vi "TS DAC Acq Stop.vi"(8 "error in (no error)":errorcluster, 11 "LNG Boiling Test Stand in":refnum<class "LNG Boiling Test Stand.lvclass">) -> (0 "error out":errorcluster, 3 "LNG Boiling Test Stand out":refnum<class "LNG Boiling Test Stand.lvclass">)   [LabVIEW 2019, in "Test Stands.lvlib" / "LNG Boiling Test Stand.lvclass"]
uses:
  LNG Boiling Test Stand.lvclass
  LNG Boiling Test Stand.lvclass/LNG Boiling Test Stand.ctl
  <vilib>/DAQmx/write.llb/DAQmx Write (Analog DBL 1Chan 1Samp).vi
  <vilib>/DAQmx/miscellaneous.llb/DAQmx Fill In Error Info.vi
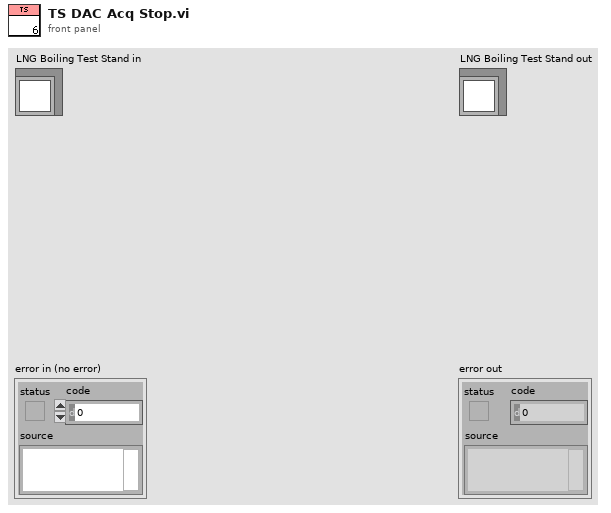
[diagram p1: front panel]
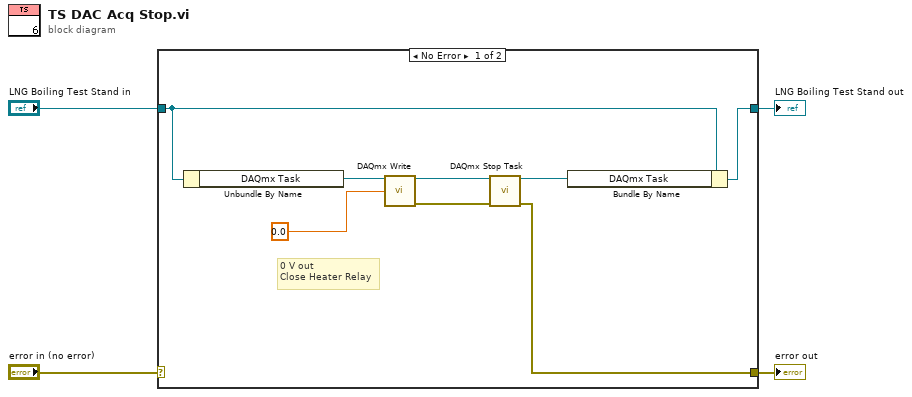
[diagram p0: block diagram]
diagram:
  n1 = case shown="No Error" "error in (no error)" {
    selector: "error in (no error)" -> [_ w14]
    tunnel: [w8 w14] -> w1
    tunnel: [w5 w13] -> w3
    tunnel: "LNG Boiling Test Stand in" -> [w7 w13]
    frame No Error {
      # "0 V out\nClose Heater Relay"
      n2 = Unbundle By Name(w7) -> ("DAQmx Task"=w11:refnum<k21>)
      n3 = call-poly <vilib>:"DAQmx Write.vi"("task/channels in"=w11, "data"=0.0) -> ("task out"=w10:refnum<k21>, "error out"=w9:errorcluster)  [unwired: 11 in, 1 out]
      n4 = call <vilib>:"DAQmx Stop Task.vi"("task/channels in"=w10, "error in"=w9) -> ("task out"=w6:refnum<k21>, "error out"=w8:errorcluster)  [unwired: 12 in]
      n5 = Bundle By Name(cluster=w7, "DAQmx Task"=w6) -> (w5:refnum<class "LNG Boiling Test Stand.lvclass">)
    }
    frame Error {
    }
  }
  "error out" <- w1
  "LNG Boiling Test Stand out" <- w3
